vi "Get Array Values (String).vi"(8 "error in (no error)":errorcluster, 11 "JSON Array in":refnum<class "JSON Array.lvclass">) -> (0 "error out":errorcluster, 2 "Strings":string[](array[string]), 3 "JSON Array out":refnum<class "JSON Array.lvclass">)   [LabVIEW 2017]
uses:
  JSON String/JSON String.lvclass
  JSON Array.lvclass
  C:/Users/tblair/Documents/Git Projects/LVJSON/Source/JSON Data Classes/JSON Structured Type/JSON Structured Type.lvclass
  C:/Users/tblair/Documents/Git Projects/LVJSON/Source/JSON Data Classes/JSON Datatype/JSON Datatype.lvclass
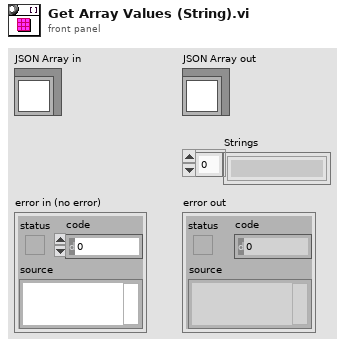
[diagram p1: front panel]
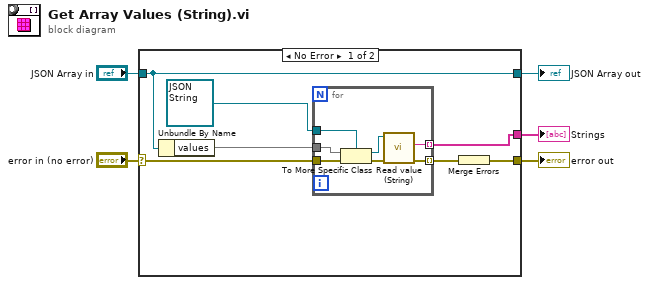
[diagram p0: block diagram]
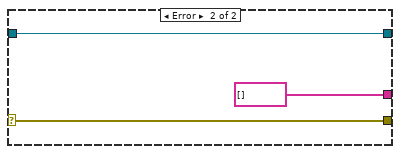
[diagram p2: hidden frame]
diagram:
  n1 = case shown="No Error" "error in (no error)" {
    selector: "error in (no error)" -> [w11 w22]
    tunnel: [w10 w22] -> w4
    tunnel: [w9 w21] -> w2
    tunnel: "JSON Array in" -> [w9 w21]
    tunnel: [w12 string[] []] -> w1
    frame No Error {
      n2 = Unbundle By Name(w9) -> ("values"=w8)
      n3 = for {
        tunnel: w8 -> [w19]
        tunnel: refnum<class "JSON String.lvclass"> refnum ("target class") -> [w18]
        tunnel: [w16] -> w12 mode=indexing
        tunnel: w11 -> [w15]
        tunnel: [w13] -> w6 mode=indexing
        n4 = To More Specific Class(target class=w18, reference=w19, error in=w15) -> (specific class reference=w17:refnum<class "JSON String.lvclass">, error out=w14:errorcluster)
        n5 = call "Read value (String).vi"("error in (no error)"=w14, "JSON String in"=w17) -> ("error out"=w13:errorcluster, "value"=w16:string)  [unwired: 7 in, 1 out]
      }
      n6 = Merge Errors(w6) -> (w10:errorcluster)
    }
    frame Error {
    }
  }
  "error out" <- w4
  "JSON Array out" <- w2
  "Strings" <- w1
